vi "6-1 글꼴설정.vi"() -> ()   [LabVIEW 2014]
uses:
  System.Windows.Forms
  System.Drawing
panel:
  out "Color":u32(colorbox) caption="색"
  out "Size":sgl
  out "Name":string
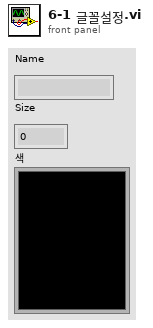
[diagram p1: front panel]
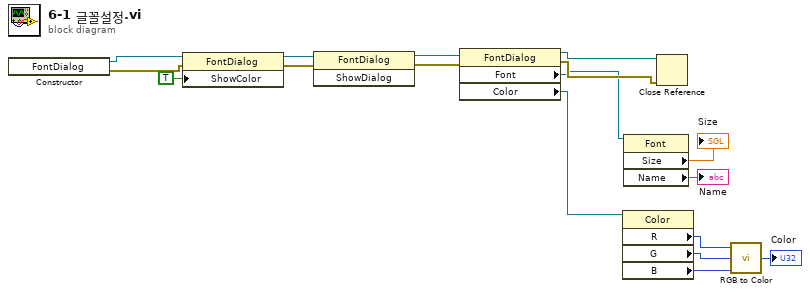
[diagram p0: block diagram]
diagram:
  n1 = constructor class="FontDialog"() -> (reference out=w17:refnum<k24>, error out=w13:errorcluster)  [unwired: 3 in, 1 out]
  n2 = property class="FontDialog"(reference=w17, error in=w13, "ShowColor"=TRUE) -> (reference out=w16:refnum<k24>, error out=w12:errorcluster)
  n3 = invoke class="FontDialog" method="ShowDialog"(reference=w16, error in=w12) -> (reference out=w15:refnum<k24>, error out=w11:errorcluster)  [unwired: 1 in, 1 out]
  n4 = property class="FontDialog"(reference=w15, error in=w11) -> (reference out=w14:refnum<k24>, error out=w10:errorcluster, "Font"=w8:refnum<k24>, "Color"=w5:refnum<k24>)
  n5 = property class="Color"(reference=w5) -> ("R"=w4:u8, "G"=w3:u8, "B"=w2:u8)  [unwired: 1 in, 2 out]
  n6 = property class="Font"(reference=w8) -> ("Size"=→"Size":sgl, "Name"=→"Name":string)  [unwired: 1 in, 2 out]
  n7 = Close Reference(reference=w14, error in (no error)=w10) -> ()  [unwired: 1 out]
  n8 = call <vilib>:"RGB to Color.vi"("B"=w2, "G"=w3, "R"=w4) -> ("Color"=→"Color":u32)
